vi "メイン.vi"() -> (2 "測定周期/ms":dbl, 3 "値転記用配列":T2[](array[typedef]) {"測定モード" items=["単発測定モード", "連続測定モード", "多点測定モード"]})   [LabVIEW 2021]
uses:
  <vilib>/Utility/miscctls.llb/LVPointTypeDef.ctl
  <vilib>/Utility/config.llb/Read Key (String).vi
  <vilib>/Utility/config.llb/Read Key (U32).vi
  <vilib>/Utility/config.llb/Read Key (I32).vi
  <vilib>/Utility/config.llb/Read Key (Boolean).vi
  <vilib>/Utility/config.llb/Read Key (Path).vi
  <vilib>/Utility/file.llb/Write Delimited Spreadsheet (string).vi
  <vilib>/Utility/config.llb/NI_LVConfig.lvlib
panel:
  in  "csv作成表_csv書込_リセット用":string[][](table)
  in  "csv作成表_リセット用":string[][](table)
  in  "csv作成表_csv書込":string[][](table)
  out "空白列カウント":dbl
  out "空白列カウント 2":dbl
  out "書込周期/ms":dbl
  out "書込CSV時間":string
  out "書込CSV日付":string
  out "書込時間":string
  out "書込日付":string
  in  "CSV保存名":string
  out "メインON/OFF_\n設定 12":T1
  out "メインON/OFF_\n保存確認 12":T1
  out "メインON/OFF_\n設定 11":T1
  out "メインON/OFF_\n保存確認 11":T1
  out "メインON/OFF_\n設定 10":T1
  out "メインON/OFF_\n保存確認 10":T1
  out "メインON/OFF_\n設定 9":T1
  out "メインON/OFF_\n保存確認 9":T1
  out "メインON/OFF_\n設定 8":T1
  out "メインON/OFF_\n保存確認 8":T1
  out "メインON/OFF_\n設定 7":T1
  out "メインON/OFF_\n保存確認 7":T1
  out "メインON/OFF_\n設定 6":T1
  out "メインON/OFF_\n保存確認 6":T1
  out "メインON/OFF_\n設定 5":T1
  out "メインON/OFF_\n保存確認 5":T1
  out "メインON/OFF_\n設定 4":T1
  out "メインON/OFF_\n保存確認 4":T1
  out "メインON/OFF_\n保存確認 3":T1
  out "メインON/OFF_\n設定 3":T1
  out "多点測定転記用配列":T2[](array[typedef]) {"測定モード" items=["単発測定モード", "連続測定モード", "多点測定モード"]}
  out "MAX/MINグローバルリセット用":string[][](array[string])
  out "メインON/OFF_\n保存確認 2":T1
  out "メインON/OFF_\n保存確認 1":T1
  out "前回値転記用配列":T2[](array[typedef]) {"測定モード" items=["単発測定モード", "連続測定モード", "多点測定モード"]}
  out "メインON/OFF_\n設定 2":T1
  in  "CSV保存先フォルダ":path
  out "G_メイン測定キャンセルボタン":bool
  out "保存ブール":bool
  out "csv作成表":string[][](table)
  out "iniフォルダパス取得":path
  out "setup.iniエラーout":errorcluster caption="エラー入力（エラーなし）"
  in  "setup.iniエラーin":errorcluster caption="エラー入力（エラーなし）"
  out "キューエラー出力":errorcluster caption="エラー出力"
  out "メイン設定_実測定から転記":T2 {"測定モード" items=["単発測定モード", "連続測定モード", "多点測定モード"]}
  in  "TOPページへ":bool caption="設定"
  out "メイン_品番品名":cluster{"品名":string, "品番前":string, "品番後":string}
  out "メインON/OFF_\n設定 1":T1
  in  "保存せずに":bool caption="設定"
  in  "保存して終了":bool caption="設定"
  out "CSV保存先":path
  in  "csv入力項目max 12":string
  in  "csv入力項目min 12":string
  in  "csv入力項目max 11":string
  in  "csv入力項目min 11":string
  in  "csv入力項目max 10":string
  in  "csv入力項目min 10":string
  in  "csv入力項目max 9":string
  in  "csv入力項目min 9":string
  in  "csv入力項目max 8":string
  in  "csv入力項目min 8":string
  in  "csv入力項目max 7":string
  in  "csv入力項目min 7":string
  in  "csv入力項目max 6":string
  in  "csv入力項目min 6":string
  in  "csv入力項目max 5":string
  in  "csv入力項目min 5":string
  in  "csv入力項目max 4":string
  in  "csv入力項目min 4":string
  in  "csv入力項目max 3":string
  in  "csv入力項目min 3":string
  in  "csv入力項目max 2":string
  in  "csv入力項目min 2":string
  in  "csv入力項目min 1":string
  in  "csv入力項目max 1":string
  in  "CSV項目名 12":T3
  in  "CSV項目名 11":T3
  in  "CSV項目名 10":T3
  in  "CSV項目名 9":T3
  in  "CSV項目名 8":T3
  in  "CSV項目名 7":T3
  in  "CSV項目名 6":T3
  in  "CSV項目名 5":T3
  in  "CSV項目名 4":T3
  in  "CSV項目名 3":T3
  in  "CSV項目名 2":T3
  in  "CSV項目名 1":T3
  out "測定新値 12":bool
  out "測定旧値 12":bool
  out "測定新値\nリセット用 12":bool
  in  "キャンセルボタン 12":T4
  in  "メインON/OFF_制御器 12":T1
  out "メイン設定No_設定 12":T5
  out "メイン設定_設定 12":T2 {"測定モード" items=["単発測定モード", "連続測定モード", "多点測定モード"]}
  in  "メイン測定ボタン_連続 12":T6
  in  "メイン測定ボタン_単発 12":T7
  out "測定新値 11":bool
  out "測定旧値 11":bool
  out "測定新値\nリセット用 11":bool
  in  "キャンセルボタン 11":T4
  in  "メインON/OFF_制御器 11":T1
  out "メイン設定No_設定 11":T5
  out "メイン設定_設定 11":T2 {"測定モード" items=["単発測定モード", "連続測定モード", "多点測定モード"]}
  in  "メイン測定ボタン_連続 11":T6
  in  "メイン測定ボタン_単発 11":T7
  out "測定新値 10":bool
  out "測定旧値 10":bool
  out "測定新値\nリセット用 10":bool
  in  "キャンセルボタン 10":T4
  in  "メインON/OFF_制御器 10":T1
  out "メイン設定No_設定 10":T5
  out "メイン設定_設定 10":T2 {"測定モード" items=["単発測定モード", "連続測定モード", "多点測定モード"]}
  in  "メイン測定ボタン_連続 10":T6
  in  "メイン測定ボタン_単発 10":T7
  out "測定新値 9":bool
  out "測定旧値 9":bool
  out "測定新値\nリセット用 9":bool
  in  "キャンセルボタン 9":T4
  in  "メインON/OFF_制御器 9":T1
  out "メイン設定No_設定 9":T5
  out "メイン設定_設定 9":T2 {"測定モード" items=["単発測定モード", "連続測定モード", "多点測定モード"]}
  in  "メイン測定ボタン_連続 9":T6
  in  "メイン測定ボタン_単発 9":T7
  out "測定新値 8":bool
  out "測定旧値 8":bool
  out "測定新値\nリセット用 8":bool
  in  "キャンセルボタン 8":T4
  in  "メインON/OFF_制御器 8":T1
  out "メイン設定No_設定 8":T5
  out "メイン設定_設定 8":T2 {"測定モード" items=["単発測定モード", "連続測定モード", "多点測定モード"]}
  in  "メイン測定ボタン_連続 8":T6
  in  "メイン測定ボタン_単発 8":T7
  out "測定新値 7":bool
  out "測定旧値 7":bool
  out "測定新値\nリセット用 7":bool
  in  "キャンセルボタン 7":T4
  in  "メインON/OFF_制御器 7":T1
  out "メイン設定No_設定 7":T5
  out "メイン設定_設定 7":T2 {"測定モード" items=["単発測定モード", "連続測定モード", "多点測定モード"]}
  in  "メイン測定ボタン_連続 7":T6
  in  "メイン測定ボタン_単発 7":T7
  out "測定新値 6":bool
  out "測定旧値 6":bool
  out "測定新値\nリセット用 6":bool
  in  "キャンセルボタン 6":T4
  in  "メインON/OFF_制御器 6":T1
  out "メイン設定No_設定 6":T5
  out "メイン設定_設定 6":T2 {"測定モード" items=["単発測定モード", "連続測定モード", "多点測定モード"]}
  in  "メイン測定ボタン_連続 6":T6
  in  "メイン測定ボタン_単発 6":T7
  out "測定新値 5":bool
  out "測定旧値 5":bool
  out "測定新値\nリセット用 5":bool
  in  "キャンセルボタン 5":T4
  in  "メインON/OFF_制御器 5":T1
  out "メイン設定No_設定 5":T5
  out "メイン設定_設定 5":T2 {"測定モード" items=["単発測定モード", "連続測定モード", "多点測定モード"]}
  in  "メイン測定ボタン_連続 5":T6
  in  "メイン測定ボタン_単発 5":T7
  out "測定新値 4":bool
  out "測定旧値 4":bool
  out "測定新値\nリセット用 4":bool
  in  "キャンセルボタン 4":T4
  in  "メインON/OFF_制御器 4":T1
  out "メイン設定No_設定 4":T5
  out "メイン設定_設定 4":T2 {"測定モード" items=["単発測定モード", "連続測定モード", "多点測定モード"]}
  in  "メイン測定ボタン_連続 4":T6
  in  "メイン測定ボタン_単発 4":T7
  out "測定新値 3":bool
  out "測定新値\nリセット用 3":bool
  out "測定旧値 3":bool
  in  "キャンセルボタン 3":T4
  in  "メインON/OFF_制御器 3":T1
  out "メイン設定No_設定 3":T5
  out "メイン設定_設定 3":T2 {"測定モード" items=["単発測定モード", "連続測定モード", "多点測定モード"]}
  in  "メイン測定ボタン_連続 3":T6
  in  "メイン測定ボタン_単発 3":T7
  out "測定新値\nリセット用 2":bool
  out "測定新値\nリセット用 1":bool
  out "測定新値 2":bool
  out "測定旧値 2":bool
  out "測定新値 1":bool
  out "測定旧値 1":bool
  in  "キャンセルボタン 2":T4
  in  "メインON/OFF_制御器 2":T1
  out "メイン設定No_設定 2":T5
  out "メイン設定_設定 2":T2 {"測定モード" items=["単発測定モード", "連続測定モード", "多点測定モード"]}
  in  "メイン測定ボタン_連続 2":T6
  in  "メイン測定ボタン_単発 2":T7
  in  "メイン測定ボタン_単発 1":T7
  in  "メインON/OFF_制御器 1":T1
  in  "キャンセルボタン 1":T4
  out "メイン設定_設定 1":T2 {"測定モード" items=["単発測定モード", "連続測定モード", "多点測定モード"]}
  in  "メイン測定ボタン_連続 1":T6
  out "メイン設定No_設定 1":T5
  # "測定データ収集"
  # "使用"
  # "規格"
  # "上限"
  # "同時測定"
  # "値クリア"
  # "No."
  # "品質チェック項目"
  # "値"
  # "測定ボタン"
  # "ボタン"
  # "ON/OFF"
  # "単位"
  # "下限"
  # "グループNo."
  # "-"
  # "品番"
  # "品名"
  # "現在測定"
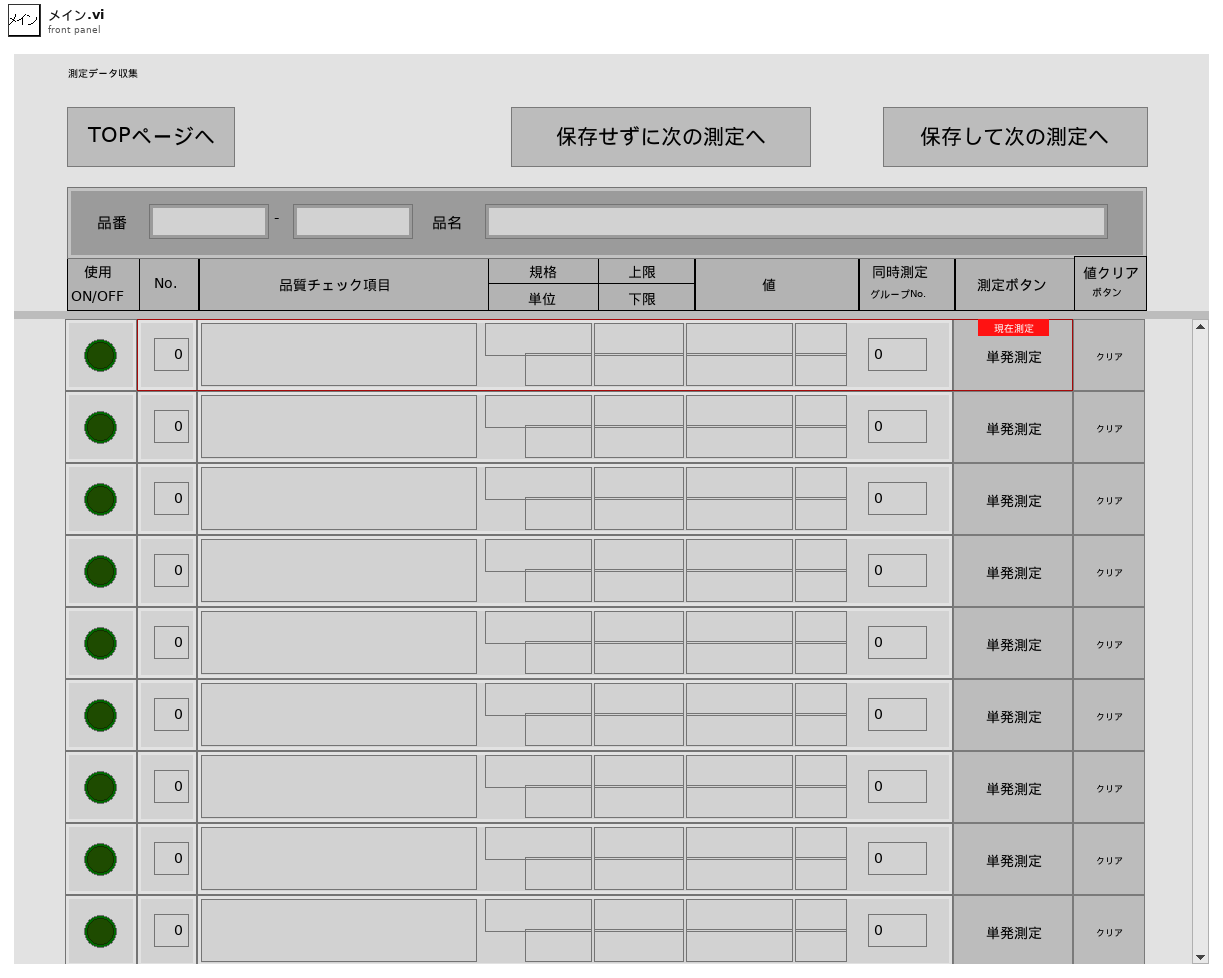
[diagram p1: front panel]
types:
  T1 = typedef "ONOFFボタン制御器.ctl" = cluster{"使用ON/OFF":bool}
  T2 = typedef "設定全項目制御器.ctl" = cluster{"規格":string, "規格上限":string, "規格下限":string, "ポートNo.":dbl, "測定モード":u16, "規格単位":string, "品質チェック項目":string, "測定周期":dbl, "実測値MAX":string, "実測値MIN":string, "実測値(MAX)":string, "実測値(MIN)":string, "測定画面表示ボタン":bool, "ゲージポートNo":refnum<visa-resource-name>}
  T3 = typedef "CSV項目名入力.ctl" = cluster{"CSV項目名":string}
  T4 = typedef "キャンセルボタン制御器.ctl" = bool
  T5 = typedef "CH設定表示器.ctl" = cluster{"No. ":dbl}
  T6 = typedef "測定ボタン制御器.ctl" = bool
  T7 = typedef "単発測定ボタン制御器.ctl" = bool
  T8 = enum8{"Enabled", "Disabled", "Disabled and Grayed Out"}
  T9 = typedef "LVPointTypeDef.ctl" = cluster{"Horizontal":i16, "Vertical":i16}
  T10 = typedef "NI_LVConfig.lvlib/Config Data RefNum.ctl" = refnum<k1>
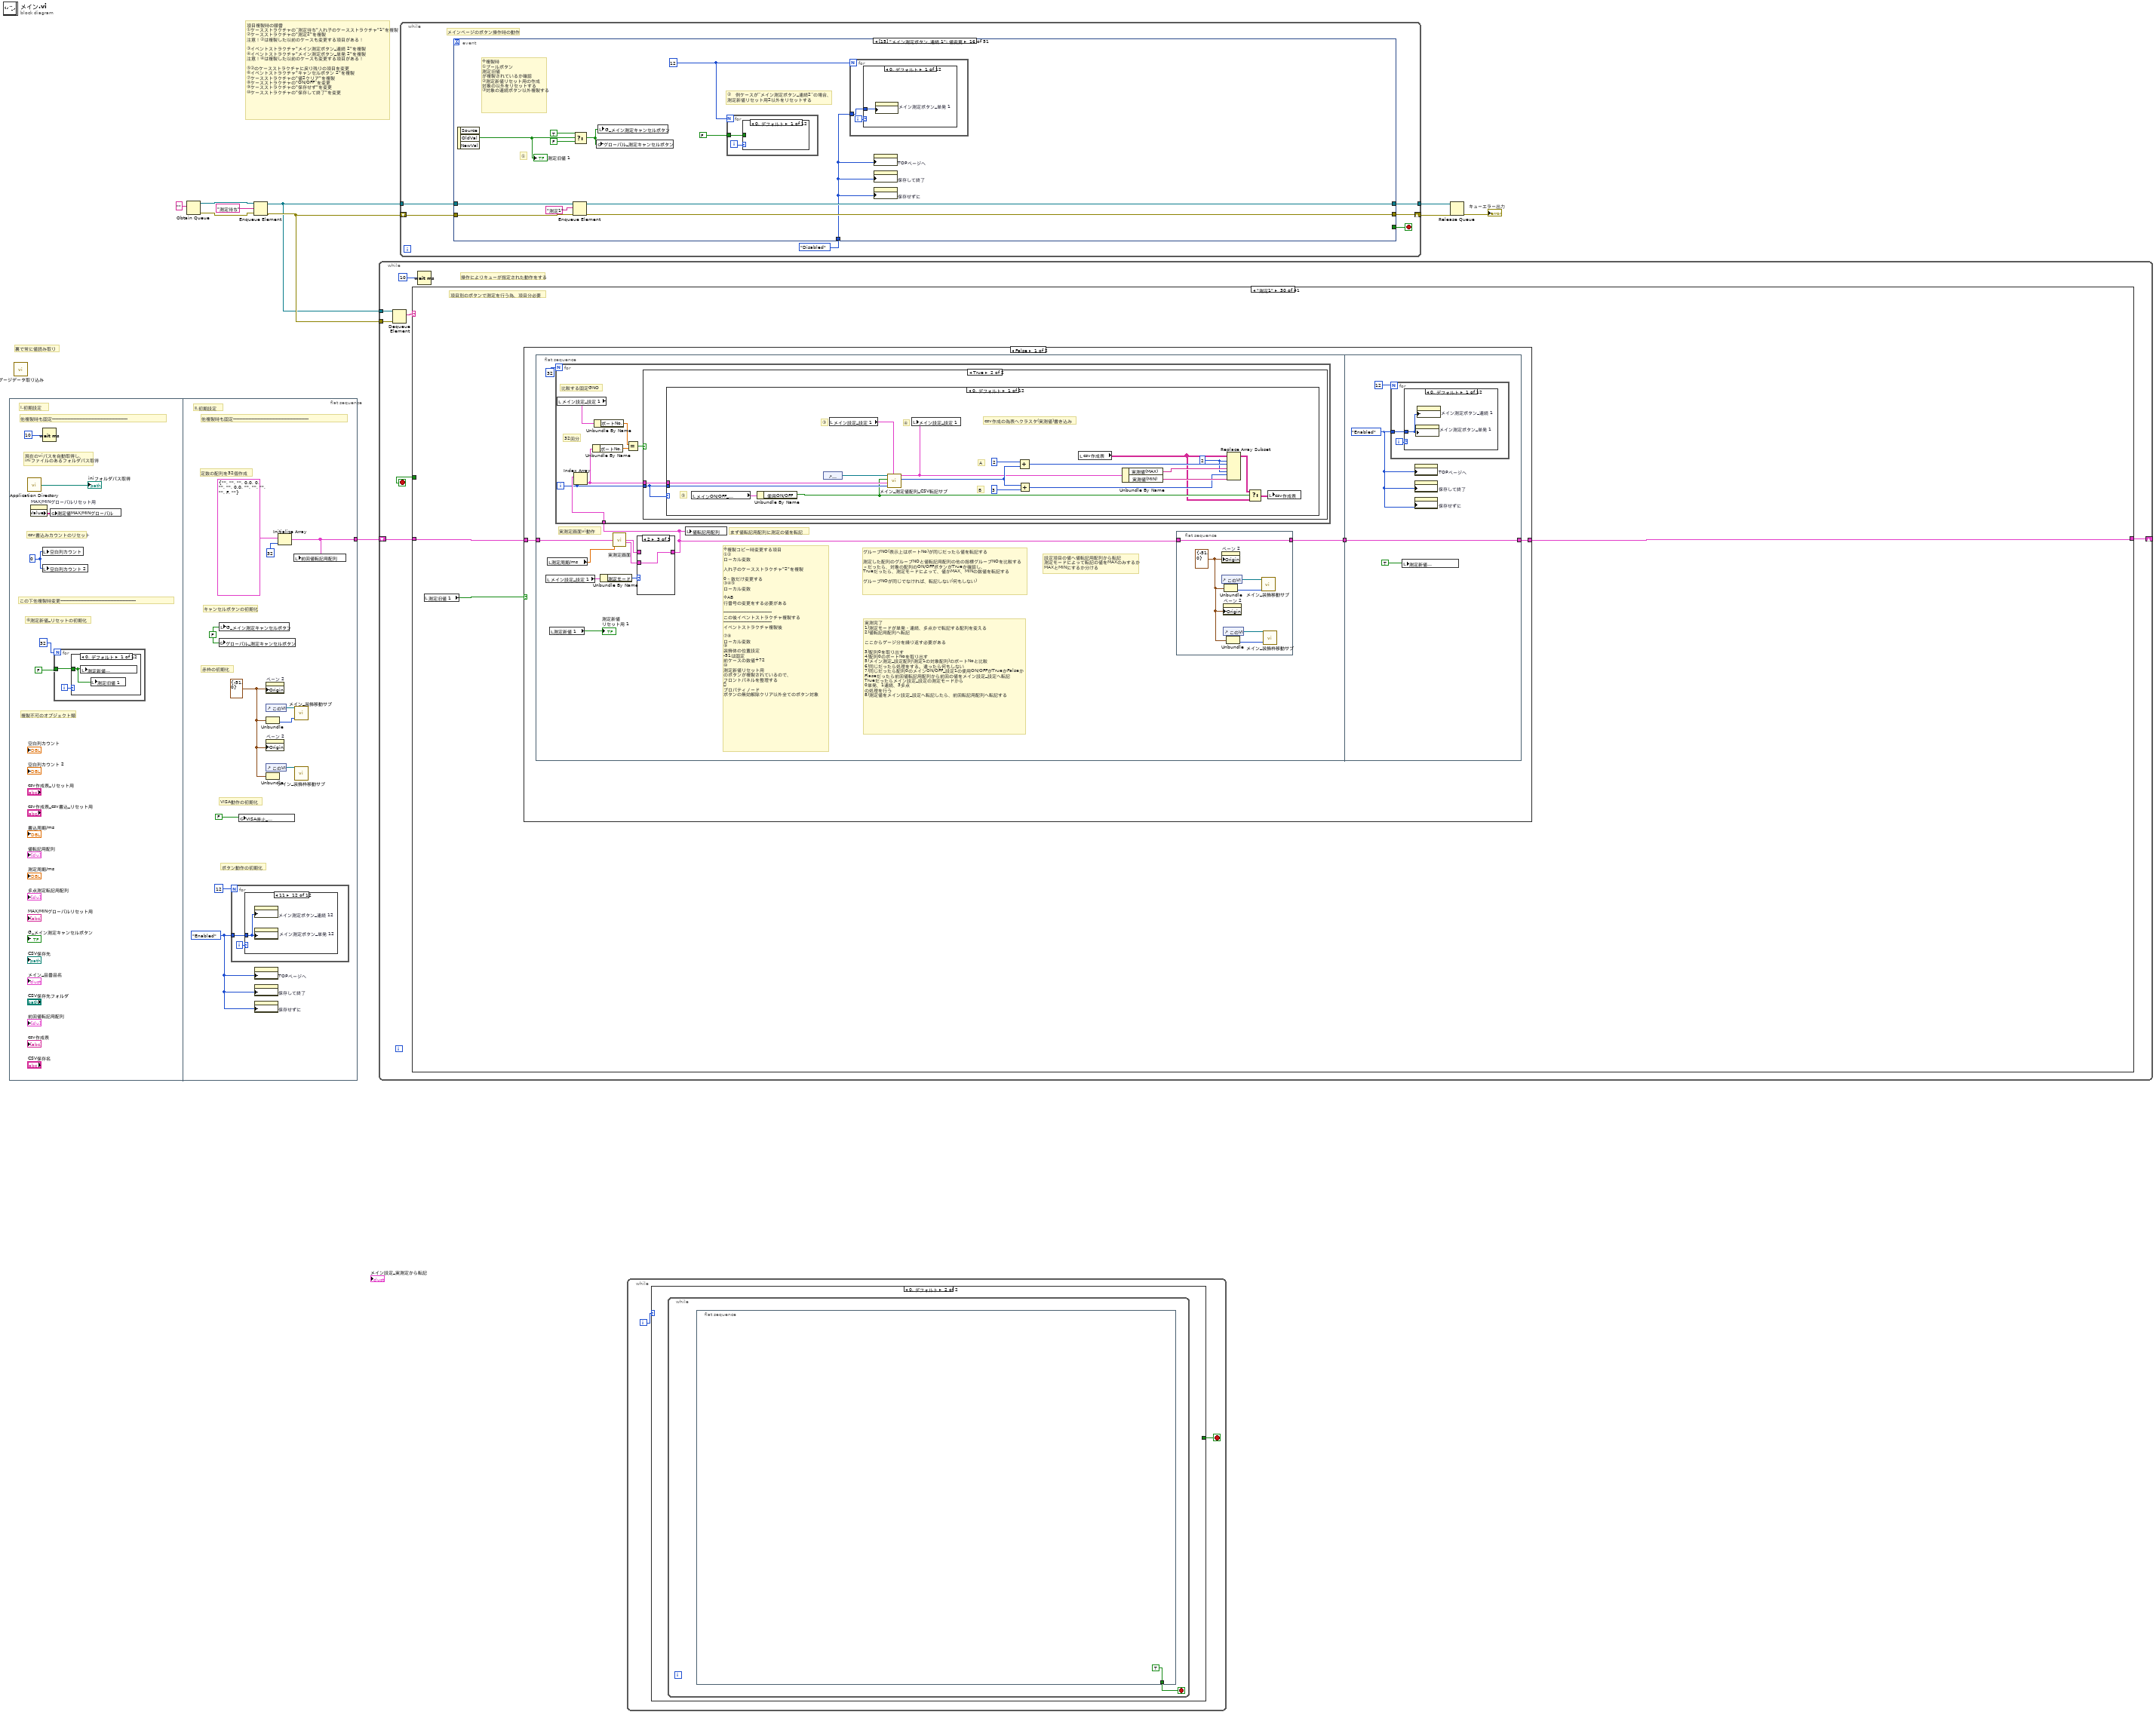
[diagram p0: block diagram]
diagram:
  # "裏で常に値読み取り"
  # "項目複製時の順番\n①ケースストラクチャの”測定待ち\"入れ子のケースストラクチャ\"1\"を複製\n②ケースストラクチャの\"測定2\"を複製\n注意！②は複製した以前のケースも変更する項目がある！\n\n③イベントストラクチャ\"メイン測定ボタン_連続 2\"を複製\n④イベントストラクチャ\"メイン測定ボタン_単発 2\"を複製\n注意！④は複製した以前のケースも変更する項目がある！\n\n⑤②のケースストラクチャに戻り残りの項目を変更\n⑥イベントストラクチャ\"キャンセルボタン 2\"を複製\n⑦ケースストラクチャの\"値2クリア\"を複製\n⑧ケースストラクチャの\"ON/OFF”を変更\n⑨ケースストラクチャの\"保存せず\"を変更\n⑩ケースストラクチャの\"保存して終了\"を変更"
  n1 = flat-sequence {
    tunnel: [w39] -> w3
    frame #0 {
      w11 = 0
      # "csv書込みカウントのリセット"
      # "現在のviパスを自動取得し、\niniファイルのあるフォルダパス取得"
      # "複製不可のオブジェクト類"
      # "この下他複製時変更--------------------------------------------------"
      # "他複製時も固定--------------------------------------------------"
      # "⑥測定新値_リセットの初期化"
      # "Ⅰ.初期設定"
      n2 = call <vilib>:"Application Directory.vi"() -> ("Application Directory"=→"iniフォルダパス取得":path)
      n3 = property on="MAX/MINグローバルリセット用" class="Arr (指定)"() -> ("Value"=w16:string[][])  [unwired: 2 in, 2 out]
      n4 = local write "空白列カウント"(w11) -> ()
      n5 = local write "空白列カウント 2"(w11) -> ()
      n6 = Wait (ms)(milliseconds to wait=10) -> ()  [unwired: 1 out]
      n7 = global write "測定値MAXMIN_G.vi" "測定値MAX/MINグローバル"(w16) -> ()
      n8 = for {
        N: 32 -> [_]
        tunnel: FALSE -> [w17]
        i -> [w18]
        n9 = case shown="0, デフォルト" w18 {
          tunnel: w17 -> [w19 w20 w21 w22 w23 w24 w25 w26 w27 w28 w29 w30]
          frame 0, Default {
            n10 = local write "測定新値\nリセット用 1"(w19) -> ()
            n11 = local write "測定旧値 1"(w19) -> ()
          }
          frame 1 {
            n12 = local write "測定新値\nリセット用 2"(w20) -> ()
            n13 = local write "測定旧値 2"(w20) -> ()
          }
          frame 2 {
            n14 = local write "測定新値\nリセット用 3"(w21) -> ()
            n15 = local write "測定旧値 3"(w21) -> ()
          }
          frame 3 {
            n16 = local write "測定新値\nリセット用 4"(w22) -> ()
            n17 = local write "測定旧値 4"(w22) -> ()
          }
          frame 4 {
            n18 = local write "測定新値\nリセット用 5"(w23) -> ()
            n19 = local write "測定旧値 5"(w23) -> ()
          }
          frame 5 {
            n20 = local write "測定新値\nリセット用 6"(w24) -> ()
            n21 = local write "測定旧値 6"(w24) -> ()
          }
          frame 6 {
            n22 = local write "測定新値\nリセット用 7"(w25) -> ()
            n23 = local write "測定旧値 7"(w25) -> ()
          }
          frame 7 {
            n24 = local write "測定新値\nリセット用 8"(w26) -> ()
            n25 = local write "測定旧値 8"(w26) -> ()
          }
          frame 8 {
            n26 = local write "測定新値\nリセット用 9"(w27) -> ()
            n27 = local write "測定旧値 9"(w27) -> ()
          }
          frame 9 {
            n28 = local write "測定新値\nリセット用 10"(w28) -> ()
            n29 = local write "測定旧値 10"(w28) -> ()
          }
          frame 10 {
            n30 = local write "測定新値\nリセット用 11"(w29) -> ()
            n31 = local write "測定旧値 11"(w29) -> ()
          }
          frame 11 {
            n32 = local write "測定新値\nリセット用 12"(w30) -> ()
            n33 = local write "測定旧値 12"(w30) -> ()
          }
        }
      }
    }
    frame #1 {
      w33 = T8."Enabled" ("無効")
      w34 = T9 {"Horizontal"=-51, "Vertical"=0} ("座標 1")
      w38 = FALSE
      # "VISA動作の初期化"
      # "ボタン動作の初期化"
      # "赤枠の初期化"
      # "キャンセルボタンの初期化"
      # "他複製時も固定--------------------------------------------------"
      # "Ⅱ.初期設定"
      # "定数の配列を32個作成"
      n34 = global write "測定キャンセルボタン.vi" "グローバル_測定キャンセルボタン"(w38) -> ()
      n35 = local write "G_メイン測定キャンセルボタン"(w38) -> ()
      n36 = for {
        N: 12 -> [_]
        tunnel: w33 -> [w42]
        i -> [w43]
        n37 = case shown="11" w43 {
          tunnel: w42 -> [w44 w45 w46 w47 w48 w49 w50 w51 w52 w53 w54 w55]
          frame 0, Default {
            n38 = property on="メイン測定ボタン_単発 1" class="Bool (指定)"("DisabledEnum"=w44) -> ()  [unwired: 2 in, 2 out]
            n39 = property on="メイン測定ボタン_連続 1" class="Bool (指定)"("DisabledEnum"=w44) -> ()  [unwired: 2 in, 2 out]
          }
          frame 1 {
            n40 = property on="メイン測定ボタン_単発 2" class="Bool (指定)"("DisabledEnum"=w45) -> ()  [unwired: 2 in, 2 out]
            n41 = property on="メイン測定ボタン_連続 2" class="Bool (指定)"("DisabledEnum"=w45) -> ()  [unwired: 2 in, 2 out]
          }
          frame 2 {
            n42 = property on="メイン測定ボタン_単発 3" class="Bool (指定)"("DisabledEnum"=w46) -> ()  [unwired: 2 in, 2 out]
            n43 = property on="メイン測定ボタン_連続 3" class="Bool (指定)"("DisabledEnum"=w46) -> ()  [unwired: 2 in, 2 out]
          }
          frame 3 {
            n44 = property on="メイン測定ボタン_単発 4" class="Bool (指定)"("DisabledEnum"=w47) -> ()  [unwired: 2 in, 2 out]
            n45 = property on="メイン測定ボタン_連続 4" class="Bool (指定)"("DisabledEnum"=w47) -> ()  [unwired: 2 in, 2 out]
          }
          frame 4 {
            n46 = property on="メイン測定ボタン_単発 5" class="Bool (指定)"("DisabledEnum"=w48) -> ()  [unwired: 2 in, 2 out]
            n47 = property on="メイン測定ボタン_連続 5" class="Bool (指定)"("DisabledEnum"=w48) -> ()  [unwired: 2 in, 2 out]
          }
          frame 5 {
            n48 = property on="メイン測定ボタン_連続 6" class="Bool (指定)"("DisabledEnum"=w49) -> ()  [unwired: 2 in, 2 out]
            n49 = property on="メイン測定ボタン_単発 6" class="Bool (指定)"("DisabledEnum"=w49) -> ()  [unwired: 2 in, 2 out]
          }
          frame 6 {
            n50 = property on="メイン測定ボタン_連続 7" class="Bool (指定)"("DisabledEnum"=w50) -> ()  [unwired: 2 in, 2 out]
            n51 = property on="メイン測定ボタン_単発 7" class="Bool (指定)"("DisabledEnum"=w50) -> ()  [unwired: 2 in, 2 out]
          }
          frame 7 {
            n52 = property on="メイン測定ボタン_単発 8" class="Bool (指定)"("DisabledEnum"=w51) -> ()  [unwired: 2 in, 2 out]
            n53 = property on="メイン測定ボタン_連続 8" class="Bool (指定)"("DisabledEnum"=w51) -> ()  [unwired: 2 in, 2 out]
          }
          frame 8 {
            n54 = property on="メイン測定ボタン_単発 9" class="Bool (指定)"("DisabledEnum"=w52) -> ()  [unwired: 2 in, 2 out]
            n55 = property on="メイン測定ボタン_連続 9" class="Bool (指定)"("DisabledEnum"=w52) -> ()  [unwired: 2 in, 2 out]
          }
          frame 9 {
            n56 = property on="メイン測定ボタン_単発 10" class="Bool (指定)"("DisabledEnum"=w53) -> ()  [unwired: 2 in, 2 out]
            n57 = property on="メイン測定ボタン_連続 10" class="Bool (指定)"("DisabledEnum"=w53) -> ()  [unwired: 2 in, 2 out]
          }
          frame 10 {
            n58 = property on="メイン測定ボタン_単発 11" class="Bool (指定)"("DisabledEnum"=w54) -> ()  [unwired: 2 in, 2 out]
            n59 = property on="メイン測定ボタン_連続 11" class="Bool (指定)"("DisabledEnum"=w54) -> ()  [unwired: 2 in, 2 out]
          }
          frame 11 {
            n60 = property on="メイン測定ボタン_連続 12" class="Bool (指定)"("DisabledEnum"=w55) -> ()  [unwired: 2 in, 2 out]
            n61 = property on="メイン測定ボタン_単発 12" class="Bool (指定)"("DisabledEnum"=w55) -> ()  [unwired: 2 in, 2 out]
          }
        }
      }
      n62 = global write "VISA停止_G.vi" "VISA停止_\nグローバル"(FALSE) -> ()
      n63 = property on="TOPページへ" class="Bool"("DisabledEnum"=w33) -> ()  [unwired: 2 in, 2 out]
      n64 = property on="保存して終了" class="Bool"("DisabledEnum"=w33) -> ()  [unwired: 2 in, 2 out]
      n65 = property on="保存せずに" class="Bool"("DisabledEnum"=w33) -> ()  [unwired: 2 in, 2 out]
      n66 = property on="ペーン 2" class="Pane"("Origin"=w34) -> ()  [unwired: 2 in, 2 out]
      n67 = control-ref of="このVI"() -> (w36:refnum<vi>)
      n68 = Unbundle(w34) -> ("Vertical"=w37:i16)  [unwired: 1 out]
      n69 = property on="ペーン 2" class="Pane"("Origin"=w34) -> ()  [unwired: 2 in, 2 out]
      n70 = control-ref of="このVI"() -> (w35:refnum<vi>)
      n71 = Unbundle(w34) -> ()  [unwired: 2 out]
      n72 = Initialize Array(T2 {"規格"="", "規格上限"="", "規格下限"="", "ポートNo."=0.0, "測定モード"=0, "規格単位"="", "品質チェック項目"="", "測定周期"=0.0, "実測値MAX"="", "実測値MIN"="", "実測値(MAX)"="", "実測値(MIN)"="", "測定画面表示ボタン"=FALSE, "ゲージポートNo"=""} ("メイン設定_設定"), 32) -> (w39:T2[])
      n73 = local write "前回値転記用配列"(w39) -> ()
      n74 = call "メイン_装飾移動サブ.vi"("Y軸座標入力"=w37, "VI入力"=w36) -> ()  [unwired: 10 in]
      n75 = call "メイン_装飾枠移動サブ.vi"("VI入力"=w35) -> ()  [unwired: 11 in]
    }
  }
  n76 = call "ゲージデータ取り込み.vi"() -> ()  [unwired: 10 in, 2 out]
  n77 = Obtain Queue(element data type="") -> (queue out=w5:refnum<queue>, error out=w4:errorcluster)  [unwired: 4 in, 1 out]
  n78 = Enqueue Element(queue=w5, element="測定待ち", error in (no error)=w4) -> (queue out=w1:refnum<queue>, error out=w2:errorcluster)  [unwired: 1 in, 1 out]
  n79 = while {
    tunnel: w1 -> [w62]
    tunnel: w2 -> [w60]
    shift-right: [w58] -> _
    shift-left: w3 -> [w59]
    stop <- w56 stop-if-true
    # "操作によりキューが指定された動作をする"
    n80 = Dequeue Element(queue=w62, error in (no error)=w60) -> (element=w61:string)  [unwired: 1 in, 3 out]
    n81 = case shown="\"測定1\"" w61 {
      tunnel: w59 -> [w63 w66 w3055 w3057 w3059 w3061 w3063 w3065 w3067 w3069 w3071 w3073 w3075 w3077 _ w3090 w3147 w3377 w3382 w3387 w3392 w3397 w3402 w3407 w3412 w3417 w3422 w3427 w3432 w3435 w3704 w3973 w4242 w4511 w4780 w5049 w5318 w5587 w5856 w6125 w6394]
      tunnel: [w63 w65 w3055 w3057 w3059 w3061 w3063 w3065 w3067 w3069 w3071 w3073 w3075 w3077 _ w3090 w3147 w3377 w3382 w3387 w3392 w3397 w3402 w3407 w3412 w3417 w3422 w3427 w3432 w3436 w3705 w3974 w4243 w4512 w4781 w5050 w5319 w5588 w5857 w6126 w6395] -> w58
      tunnel: [_ _ _ _ _ _ _ _ _ _ _ _ _ _ w3079 _ _ _ _ _ _ _ _ _ _ _ _ _ _ _ _ _ _ _ _ _ _ _ _ _ _] -> w56
      frame "デフォ", Default {
      }
      frame "測定待ち" {
        # "プログラム起動時に動作"
        n82 = flat-sequence {
          tunnel: w66 -> [w68]
          tunnel: [w67] -> w64
          tunnel: [w3014] -> w65
          tunnel: w64 -> [w3014]
          frame #0 {
            n83 = while {
              shift-right: [w70] -> w67
              shift-left: w68 -> [w71]
              i -> [w81]
              stop <- w69 stop-if-true
              n84 = local read "iniフォルダパス取得"() -> (w80:path)
              n85 = Build Path "パス作成"(base path=w80, name or relative path=path "setting1.ini") -> (appended path=w79:path)
              n86 = call <vilib>:"Open Config Data.vi"("error in (no error)"="setup.iniエラーin", "configuration file path"=w79) -> ("error out"=w75:errorcluster, "refnum"=w76:T10)  [unwired: 1 in, 7 out]
              n87 = case shown="0, デフォルト" w81 {
                tunnel: w76 -> [w87 w456 w689 w922 w1155 w1388 w1621 w1854 w2087 w2320 w2553 w2787]
                tunnel: w75 -> [w86 w455 w688 w921 w1154 w1387 w1620 w1853 w2086 w2319 w2552 w2786]
                tunnel: [w85 w458 w691 w924 w1157 w1390 w1623 w1856 w2089 w2322 w2555 w2789] -> w73
                tunnel: [w84 w457 w690 w923 w1156 w1389 w1622 w1855 w2088 w2321 w2554 w2788] -> w72
                tunnel: w71 -> [w83 w454 w687 w920 w1153 w1386 w1619 w1852 w2085 w2318 w2551 w2785]
                tunnel: [w82 w453 w686 w919 w1152 w1385 w1618 w1851 w2084 w2317 w2550 w2784] -> w70
                tunnel: [_ _ _ _ _ _ _ _ _ _ _ TRUE] -> w69
                frame 0, Default {
                  n88 = while {
                    tunnel: w87 -> [w93]
                    tunnel: w86 -> [w92]
                    tunnel: [w91] -> w85
                    tunnel: [w90] -> w84
                    shift-right: [w88] -> w82
                    shift-left: w83 -> [w89]
                    stop <- w94 stop-if-true
                    n89 = flat-sequence {
                      tunnel: [TRUE] -> w94
                      tunnel: w93 -> [w110]
                      tunnel: w92 -> [w109]
                      tunnel: [w108] -> w91
                      tunnel: [w107] -> w90
                      tunnel: w89 -> [w101]
                      tunnel: [w102] -> w88
                      frame #0 {
                        w97 = T9 {"Horizontal"=-51, "Vertical"=0} ("座標 1")
                        w98 = FALSE
                        # "1つ目の配列に転記"
                        # "0、デフォルトのケースは複製不可\n複製時、設定項目の配列やボタンも複製する為、下記のボタン類の移動はしない事"
                        # "iniからデータ読み取り"
                        n90 = flat-sequence {
                          tunnel: [w117] -> w112
                          tunnel: [w116] -> w111
                          tunnel: w110 -> [w115]
                          tunnel: w109 -> [w114]
                          tunnel: w112 -> [w184]
                          tunnel: w111 -> [w185]
                          tunnel: [w182] -> w106
                          tunnel: [w183] -> w105
                          tunnel: w106 -> [w396]
                          tunnel: w105 -> [w395]
                          tunnel: [w396] -> w104
                          tunnel: [w395] -> w103
                          tunnel: [w443] -> w107
                          tunnel: [w444] -> w108
                          tunnel: w104 -> [w444]
                          tunnel: w103 -> [w443]
                          tunnel: [w440] -> w100
                          frame #0 {
                            # "setting.iniファイルからのデータ読み取り"
                            n91 = for {
                              tunnel: string[] ["品番前", "品番後", "品名", "測定周期", "CSV保存名", "書込周期"] -> [w127] mode=indexing
                              shift-right: [w126] -> w116
                              shift-left: w115 -> [w125]
                              tunnel: "品番・品名" -> [w124]
                              shift-right: [w122] -> w117
                              shift-left: w114 -> [w123]
                              i -> [w128]
                              n92 = local read "メイン_品番品名"() -> (w120:cluster{"品名":string, "品番前":string, "品番後":string})
                              n93 = case shown="5" w128 {
                                tunnel: w127 -> [w137 w146 w155 w163 w171 w179]
                                tunnel: [w136 w145 w153 w161 w169 w177] -> w126
                                tunnel: w125 -> [w135 w144 w154 w162 w170 w178]
                                tunnel: w124 -> [w134 w143 w152 w160 w168 w176]
                                tunnel: w123 -> [w133 w142 w151 w159 w167 w175]
                                tunnel: [w132 w141 w150 w158 w166 w174] -> w122
                                tunnel: [w129 w139 w148 w156 w164 w172] -> w121
                                tunnel: w120 -> [w130 w138 w147 _ _ _]
                                frame 0, Default {
                                n94 = call-poly <vilib>:"Read Key.vi"("section"=w134, "error in (no error)"=w133, "key"=w137, "refnum"=w135) -> ("error out"=w132:errorcluster, "value"=w131:string, "refnum out"=w136:T10)  [unwired: 4 in, 1 out]
                                n95 = Bundle By Name(cluster=w130, "品番前"=w131) -> (w129:cluster{"品名":string, "品番前":string, "品番後":string})
                                }
                                frame 1 {
                                n96 = call-poly <vilib>:"Read Key.vi"("section"=w143, "error in (no error)"=w142, "key"=w146, "refnum"=w144) -> ("error out"=w141:errorcluster, "value"=w140:string, "refnum out"=w145:T10)  [unwired: 4 in, 1 out]
                                n97 = Bundle By Name(cluster=w138, "品番後"=w140) -> (w139:cluster{"品名":string, "品番前":string, "品番後":string})
                                }
                                frame 2 {
                                n98 = call-poly <vilib>:"Read Key.vi"("section"=w152, "error in (no error)"=w151, "key"=w155, "refnum"=w154) -> ("error out"=w150:errorcluster, "value"=w149:string, "refnum out"=w153:T10)  [unwired: 4 in, 1 out]
                                n99 = Bundle By Name(cluster=w147, "品名"=w149) -> (w148:cluster{"品名":string, "品番前":string, "品番後":string})
                                }
                                frame 3 {
                                n100 = local read "メイン_品番品名"() -> (w156:cluster{"品名":string, "品番前":string, "品番後":string})
                                n101 = call-poly <vilib>:"Read Key.vi"("section"=w160, "error in (no error)"=w159, "key"=w163, "refnum"=w162) -> ("error out"=w158:errorcluster, "value"=w157:u32, "refnum out"=w161:T10)  [unwired: 4 in, 1 out]
                                n102 = local write "測定周期/ms"(w157) -> ()
                                }
                                frame 4 {
                                n103 = local read "メイン_品番品名"() -> (w164:cluster{"品名":string, "品番前":string, "品番後":string})
                                n104 = call-poly <vilib>:"Read Key.vi"("section"=w168, "error in (no error)"=w167, "key"=w171, "refnum"=w170) -> ("error out"=w166:errorcluster, "value"=w165:string, "refnum out"=w169:T10)  [unwired: 4 in, 1 out]
                                n105 = local write "CSV保存名"(w165) -> ()
                                }
                                frame 5 {
                                n106 = local read "メイン_品番品名"() -> (w172:cluster{"品名":string, "品番前":string, "品番後":string})
                                n107 = call-poly <vilib>:"Read Key.vi"("section"=w176, "error in (no error)"=w175, "key"=w179, "refnum"=w178) -> ("error out"=w174:errorcluster, "value"=w173:u32, "refnum out"=w177:T10)  [unwired: 4 in, 1 out]
                                n108 = local write "書込周期/ms"(w173) -> ()
                                }
                              }
                              n109 = local write "メイン_品番品名"(w121) -> ()
                            }
                          }
                          frame #1 {
                            # "setting.iniファイルからの設定項目の読み取り"
                            n110 = for {
                              shift-right: [w188] -> w182
                              shift-left: w185 -> [w189]
                              tunnel: string[] ["No."] -> [w191] mode=indexing
                              tunnel: "No." -> [w190]
                              shift-right: [w186] -> w183
                              shift-left: w184 -> [w187]
                              i -> [w192]
                              n111 = case shown="0, デフォルト" w192 {
                                tunnel: w191 -> [w211]
                                tunnel: w190 -> [w210]
                                tunnel: w189 -> [w209]
                                tunnel: [w195] -> w188
                                tunnel: w187 -> [w206]
                                tunnel: [w196] -> w186
                                frame 0, Default {
                                w194 = "設定"
                                n112 = call-poly <vilib>:"Read Key.vi"("section"=w210, "error in (no error)"=w206, "key"=w211, "refnum"=w209) -> ("error out"=w205:errorcluster, "value"=w202:i32, "refnum out"=w208:T10)  [unwired: 4 in, 1 out]
                                n113 = local read "メイン設定No_設定 1"() -> (w201:T5)
                                n114 = Bundle By Name(cluster=w201, "No."=w202) -> (w203:T5)
                                n115 = local write "メイン設定No_設定 1"(w203) -> ()
                                n116 = for {
                                shift-right: [w257] -> w207
                                shift-left: w208 -> [w259]
                                tunnel: w194 -> [w258]
                                shift-right: [w254] -> w204
                                shift-left: w205 -> [w255]
                                tunnel: string[] ["規格", "規格上限", "規格下限", "ポートNo.", "測定モード", "規格単位", "品質チェック項目", "測定周期", "実測MAX", "実測MIN", "実測(MAX)", "実測(MIN)", "測定画面表示ボタン", "ゲージポートNo."] -> [w253] mode=indexing
                                i -> [w256]
                                n117 = local read "メイン設定_設定 1"() -> (w251:T2)
                                n118 = case shown="4" w256 {
                                tunnel: w259 -> [w268 w277 w286 w295 w304 w313 w322 w331 w340 w349 w358 w367 w376 w385]
                                tunnel: [w267 w276 w285 w294 w303 w312 w321 w330 w339 w348 w357 w366 w375 w384] -> w257
                                tunnel: w258 -> [w266 w275 w284 w293 w302 w311 w320 w329 w338 w347 w356 w365 w374 w383]
                                tunnel: w255 -> [w265 w274 w283 w292 w301 w310 w319 w328 w337 w346 w355 w364 w373 w382]
                                tunnel: [w264 w273 w282 w291 w300 w309 w318 w327 w336 w345 w354 w363 w372 w381] -> w254
                                tunnel: w253 -> [_ _ _ _ _ w307 _ _ _ _ _ _ _ _]
                                tunnel: w253 -> [_ _ _ _ _ _ w316 _ _ _ _ w361 _ _]
                                tunnel: w253 -> [w262 w271 w280 w289 w298 _ _ w325 w334 w343 w352 _ w370 w379]
                                tunnel: [w261 w270 w279 w288 w297 w305 w314 w323 w333 w342 w351 w360 w369 w378] -> w252
                                tunnel: w251 -> [w260 w269 w278 w287 w296 w306 w315 w324 w332 w341 w350 w359 w368 w377]
                                frame 0, Default {
                                n119 = call-poly <vilib>:"Read Key.vi"("section"=w266, "error in (no error)"=w265, "key"=w262, "refnum"=w268) -> ("error out"=w264:errorcluster, "value"=w263:string, "refnum out"=w267:T10)  [unwired: 4 in, 1 out]
                                n120 = Bundle By Name(cluster=w260, "規格"=w263) -> (w261:T2)
                                }
                                frame 1 {
                                n121 = call-poly <vilib>:"Read Key.vi"("section"=w275, "error in (no error)"=w274, "key"=w271, "refnum"=w277) -> ("error out"=w273:errorcluster, "value"=w272:string, "refnum out"=w276:T10)  [unwired: 4 in, 1 out]
                                n122 = Bundle By Name(cluster=w269, "規格上限"=w272) -> (w270:T2)
                                }
                                frame 2 {
                                n123 = call-poly <vilib>:"Read Key.vi"("section"=w284, "error in (no error)"=w283, "key"=w280, "refnum"=w286) -> ("error out"=w282:errorcluster, "value"=w281:string, "refnum out"=w285:T10)  [unwired: 4 in, 1 out]
                                n124 = Bundle By Name(cluster=w278, "規格下限"=w281) -> (w279:T2)
                                }
                                frame 3 {
                                n125 = call-poly <vilib>:"Read Key.vi"("section"=w293, "error in (no error)"=w292, "key"=w289, "refnum"=w295) -> ("error out"=w291:errorcluster, "value"=w290:i32, "refnum out"=w294:T10)  [unwired: 4 in, 1 out]
                                n126 = Bundle By Name(cluster=w287, "ポートNo."=w290) -> (w288:T2)
                                }
                                frame 4 {
                                n127 = call-poly <vilib>:"Read Key.vi"("section"=w302, "error in (no error)"=w301, "key"=w298, "refnum"=w304) -> ("error out"=w300:errorcluster, "value"=w299:i32, "refnum out"=w303:T10)  [unwired: 4 in, 1 out]
                                n128 = Bundle By Name(cluster=w296, "測定モード"=w299) -> (w297:T2)
                                }
                                frame 5 {
                                n129 = call-poly <vilib>:"Read Key.vi"("section"=w311, "error in (no error)"=w310, "key"=w307, "refnum"=w313) -> ("error out"=w309:errorcluster, "value"=w308:string, "refnum out"=w312:T10)  [unwired: 4 in, 1 out]
                                n130 = Bundle By Name(cluster=w306, "規格単位"=w308) -> (w305:T2)
                                }
                                frame 6 {
                                n131 = call-poly <vilib>:"Read Key.vi"("section"=w320, "error in (no error)"=w319, "key"=w316, "refnum"=w322) -> ("error out"=w318:errorcluster, "value"=w317:string, "refnum out"=w321:T10)  [unwired: 4 in, 1 out]
                                n132 = Bundle By Name(cluster=w315, "品質チェック項目"=w317) -> (w314:T2)
                                }
                                frame 7 {
                                n133 = call-poly <vilib>:"Read Key.vi"("section"=w329, "error in (no error)"=w328, "key"=w325, "refnum"=w331) -> ("error out"=w327:errorcluster, "value"=w326:i32, "refnum out"=w330:T10)  [unwired: 4 in, 1 out]
                                n134 = Bundle By Name(cluster=w324, "測定周期"=w326) -> (w323:T2)
                                }
                                frame 8 {
                                n135 = call-poly <vilib>:"Read Key.vi"("section"=w338, "error in (no error)"=w337, "key"=w334, "refnum"=w340) -> ("error out"=w336:errorcluster, "value"=w335:string, "refnum out"=w339:T10)  [unwired: 4 in, 1 out]
                                n136 = Bundle By Name(cluster=w332, "実測値MAX"=w335) -> (w333:T2)
                                }
                                frame 9 {
                                n137 = call-poly <vilib>:"Read Key.vi"("section"=w347, "error in (no error)"=w346, "key"=w343, "refnum"=w349) -> ("error out"=w345:errorcluster, "value"=w344:string, "refnum out"=w348:T10)  [unwired: 4 in, 1 out]
                                n138 = Bundle By Name(cluster=w341, "実測値MIN"=w344) -> (w342:T2)
                                }
                                frame 10 {
                                n139 = call-poly <vilib>:"Read Key.vi"("section"=w356, "error in (no error)"=w355, "key"=w352, "refnum"=w358) -> ("error out"=w354:errorcluster, "value"=w353:string, "refnum out"=w357:T10)  [unwired: 4 in, 1 out]
                                n140 = Bundle By Name(cluster=w350, "実測値(MAX)"=w353) -> (w351:T2)
                                }
                                frame 11 {
                                n141 = call-poly <vilib>:"Read Key.vi"("section"=w365, "error in (no error)"=w364, "key"=w361, "refnum"=w367) -> ("error out"=w363:errorcluster, "value"=w362:string, "refnum out"=w366:T10)  [unwired: 4 in, 1 out]
                                n142 = Bundle By Name(cluster=w359, "実測値(MIN)"=w362) -> (w360:T2)
                                }
                                frame 12 {
                                n143 = call-poly <vilib>:"Read Key.vi"("section"=w374, "error in (no error)"=w373, "key"=w370, "refnum"=w376) -> ("error out"=w372:errorcluster, "value"=w371:bool, "refnum out"=w375:T10)  [unwired: 4 in, 1 out]
                                n144 = Bundle By Name(cluster=w368, "測定画面表示ボタン"=w371) -> (w369:T2)
                                }
                                frame 13 {
                                n145 = call-poly <vilib>:"Read Key.vi"("section"=w383, "error in (no error)"=w382, "key"=w379, "refnum"=w385) -> ("error out"=w381:errorcluster, "value"=w380:string, "refnum out"=w384:T10)  [unwired: 4 in, 1 out]
                                n146 = Bundle By Name(cluster=w377, "ゲージポートNo"=w380) -> (w378:T2)
                                }
                                }
                                n147 = local write "メイン設定_設定 1"(w252) -> ()
                                }
                                n148 = for {
                                shift-right: [w232] -> w197
                                shift-left: w207 -> [w230]
                                tunnel: w194 -> [w229]
                                shift-right: [w227] -> w198
                                shift-left: w204 -> [w228]
                                tunnel: string[] ["使用ON/OFF", "CSVヘッダー名"] -> [w226] mode=indexing
                                i -> [w231]
                                n149 = case shown="1" w231 {
                                tunnel: [w241 w250] -> w232
                                tunnel: w230 -> [w240 w249]
                                tunnel: w229 -> [w239 w248]
                                tunnel: w228 -> [w238 w247]
                                tunnel: [w237 w246] -> w227
                                tunnel: w226 -> [w233 w242]
                                frame 0, Default {
                                n150 = local read "メインON/OFF_\n設定 1"() -> (w234:T1)
                                n151 = call-poly <vilib>:"Read Key.vi"("section"=w239, "error in (no error)"=w238, "key"=w233, "refnum"=w240) -> ("error out"=w237:errorcluster, "value"=w236:bool, "refnum out"=w241:T10)  [unwired: 4 in, 1 out]
                                n152 = Bundle By Name(cluster=w234, "使用ON/OFF"=w236) -> (w235:T1)
                                n153 = local write "メインON/OFF_\n設定 1"(w235) -> ()
                                }
                                frame 1 {
                                n154 = local read "CSV項目名 1"() -> (w243:T3)
                                n155 = call-poly <vilib>:"Read Key.vi"("section"=w248, "error in (no error)"=w247, "key"=w242, "refnum"=w249) -> ("error out"=w246:errorcluster, "value"=w245:string, "refnum out"=w250:T10)  [unwired: 4 in, 1 out]
                                n156 = Bundle By Name(cluster=w243, "CSV項目名"=w245) -> (w244:T3)
                                n157 = local write "CSV項目名 1"(w244) -> ()
                                }
                                }
                                }
                                n158 = for {
                                tunnel: string[] ["CSV保存先フォルダ"] -> [w217] mode=indexing
                                shift-right: [w214] -> w195
                                shift-left: w197 -> [w215]
                                tunnel: w194 -> [w216]
                                shift-right: [w213] -> w196
                                shift-left: w198 -> [w212]
                                i -> [w218]
                                n159 = case shown="0, デフォルト" w218 {
                                tunnel: w217 -> [w221]
                                tunnel: w216 -> [w225]
                                tunnel: w215 -> [w222]
                                tunnel: [w224] -> w214
                                tunnel: [w223] -> w213
                                tunnel: w212 -> [w220]
                                frame 0, Default {
                                n160 = call-poly <vilib>:"Read Key.vi"("section"=w225, "error in (no error)"=w220, "key"=w221, "refnum"=w222) -> ("error out"=w223:errorcluster, "value"=w219:path, "refnum out"=w224:T10)  [unwired: 4 in, 1 out]
                                n161 = local write "CSV保存先"(w219) -> ()
                                }
                                }
                                }
                                }
                              }
                            }
                          }
                          frame #2 {
                            # "csvヘッダー項目作成"
                            n162 = local read "CSV項目名 1"() -> (w389:T3)
                            n163 = Unbundle By Name(w389) -> ("CSV項目名"=w390:string)
                            n164 = local read "メイン設定_設定 1"() -> (w394:T2)
                            n165 = Unbundle By Name(w394) -> ("測定モード"=w386:u16)
                            n166 = case shown="0, デフォルト" w386 {
                              tunnel: w390 -> [w400 w412 w424]
                              tunnel: [w398 w410 w422] -> w388
                              tunnel: [w397 w409 w421] -> w387
                              frame 1 {
                                n167 = Empty String/Path?(string/path=w400) -> (empty?=w399:bool)
                                n168 = case shown="FALSE" w399 {
                                tunnel: w400 -> [w406 _]
                                tunnel: w400 -> [w405 _]
                                tunnel: [w402 ""] -> w398
                                tunnel: [w401 ""] -> w397
                                frame False {
                                n169 = Concatenate Strings(w406, "_max") -> (w402:string)
                                n170 = Concatenate Strings(w405, "_min") -> (w401:string)
                                }
                                frame True {
                                }
                                }
                              }
                              frame 2 {
                                n171 = Empty String/Path?(string/path=w412) -> (empty?=w411:bool)
                                n172 = case shown="FALSE" w411 {
                                tunnel: w412 -> [w418 _]
                                tunnel: w412 -> [w417 _]
                                tunnel: [w414 ""] -> w410
                                tunnel: [w413 ""] -> w409
                                frame False {
                                n173 = Concatenate Strings(w418, "_max") -> (w414:string)
                                n174 = Concatenate Strings(w417, "_min") -> (w413:string)
                                }
                                frame True {
                                }
                                }
                              }
                              frame 0, Default {
                                n175 = Empty String/Path?(string/path=w424) -> (empty?=w423:bool)
                                n176 = case shown="FALSE" w423 {
                                tunnel: w424 -> [w428 _]
                                tunnel: [w426 ""] -> w422
                                tunnel: ["" ""] -> w421
                                frame False {
                                n177 = Concatenate Strings(w428, "_value") -> (w426:string)
                                }
                                frame True {
                                }
                                }
                              }
                            }
                            n178 = case shown="0, デフォルト" w386 {
                              tunnel: ["単発測定" _ "多点測定"] -> w393
                              tunnel: [FALSE TRUE FALSE] -> w392
                              tunnel: [TRUE FALSE TRUE] -> w391
                              frame 0, Default {
                              }
                              frame 1 {
                              }
                              frame 2 {
                              }
                            }
                            n179 = local write "csv入力項目min 1"(w387) -> ()
                            n180 = property on="メイン測定ボタン_単発 1" class="Bool (指定)"("BoolText.Text"=w393) -> ()  [unwired: 2 in, 2 out]
                            n181 = local write "csv入力項目max 1"(w388) -> ()
                            n182 = property on="メイン測定ボタン_単発" class="Bool (指定)"("Visible"=w391) -> ()  [unwired: 2 in, 2 out]
                            n183 = property on="メイン測定ボタン_連続 1" class="Bool (指定)"("Visible"=w392) -> ()  [unwired: 2 in, 2 out]
                          }
                          frame #3 {
                            n184 = local read "メイン設定_設定 1"() -> (w440:T2)
                            n185 = Unbundle By Name(w440) -> ("測定画面表示ボタン"=w441:bool)
                            n186 = case shown="FALSE" w441 {
                              tunnel: [w445 TRUE] -> w439
                              frame False {
